vi "1.5.10-Unique Number.vi"() -> (0 "Number":u8)   [LabVIEW 2011]
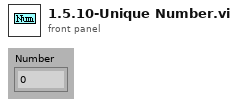
[diagram p1: front panel]
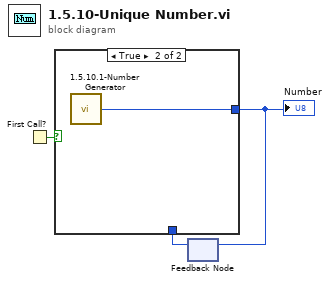
[diagram p0: block diagram]
diagram:
  n1 = First Call?() -> (First Call?: T/F=w1:bool)
  n2 = feedback #1() -> (w3:u8)  [unwired: 1 in]
  n3 = case shown="True" w1 {
    tunnel: [w4 w5] -> w2
    tunnel: w3 -> [w4 _]
    frame False {
    }
    frame True {
      n4 = call "1.5.10.1-Number Generator.vi"() -> ("Number"=w5:u8)
    }
  }
  "Number" <- w2
  n5 = feedback-in #1(w2) -> ()
